vi "processamento_dos_dados_medios_de_caracterização.vi"() -> ()   [LabVIEW 2011]
uses:
  <vilib>/Analysis/NI_AALPro.lvlib
  <vilib>/Analysis/polynomials.llb/1D Polynomial Evaluation (DBL).vi
panel:
  out "Regressão Linear":string
  out "Coeficiente de Determinação":dbl
  out "Força aplicada (N)":dbl[](array[numeric])
  out "Força calculada \n(N)":dbl[](array[numeric])
  out "Coeficientes da Regressão":dbl[](array[numeric])
  out "Tensão e Força do Sinal":cluster{"Y":dbl[], "Y":dbl[]}[](graph)
  out "Tensão elétrica \nmedida (mV/V)":dbl[](array[numeric])
  # "PROGRAMA PARA O PROCESSAMENTO DOS DADOS \nDO PROCEDIMENTO DE CARACTERIZAÇÃO"
  # "CONVERSÃO DE TENSÃO ELÉTRICA (mV/V) PARA FORÇA (N)"
  # "Desenvolvido por Eloi Antonio Triaca"
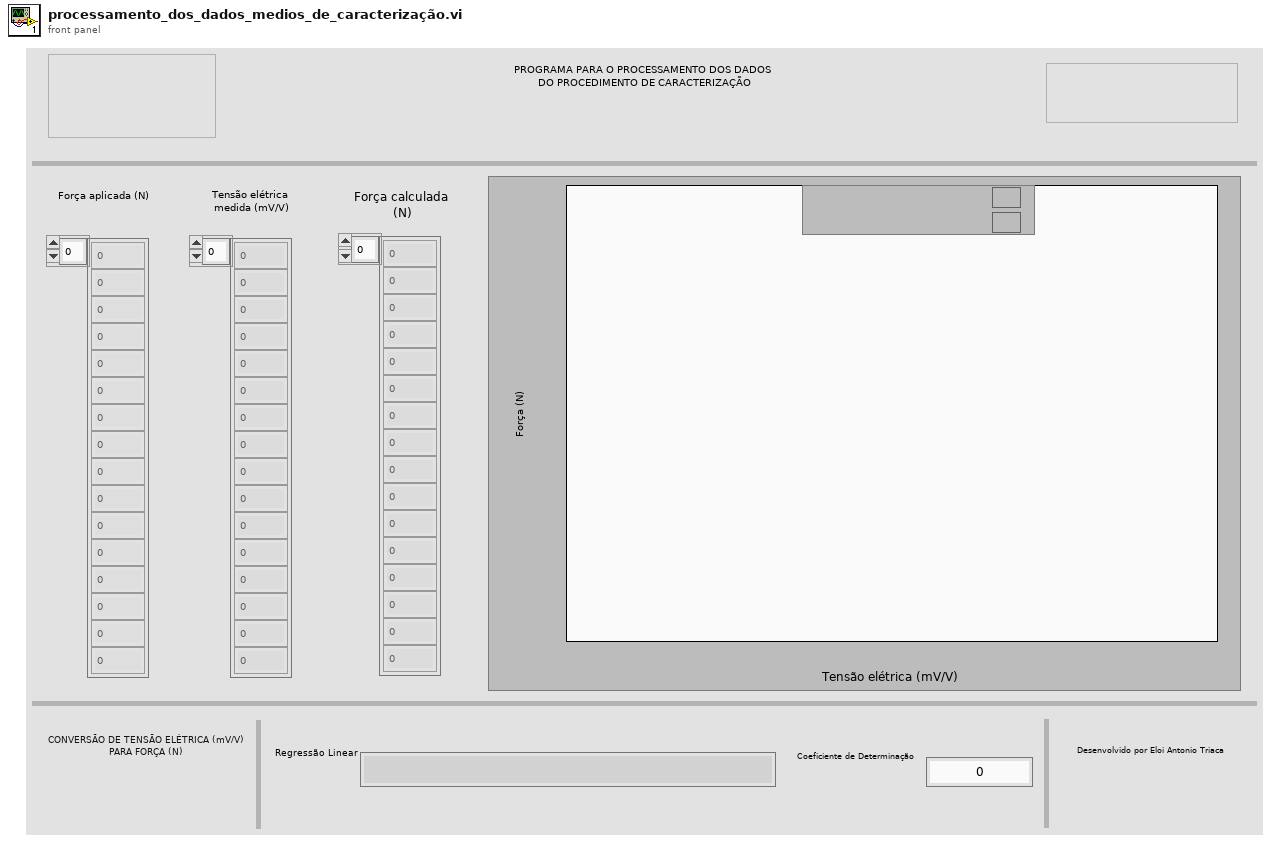
[diagram p1: front panel]
types:
  T1 = cluster{"Best Polynomial Fit":dbl[], "array":dbl[]}
  T2 = cluster{"Best Polynomial Fit":dbl[], "array":dbl[]}[]
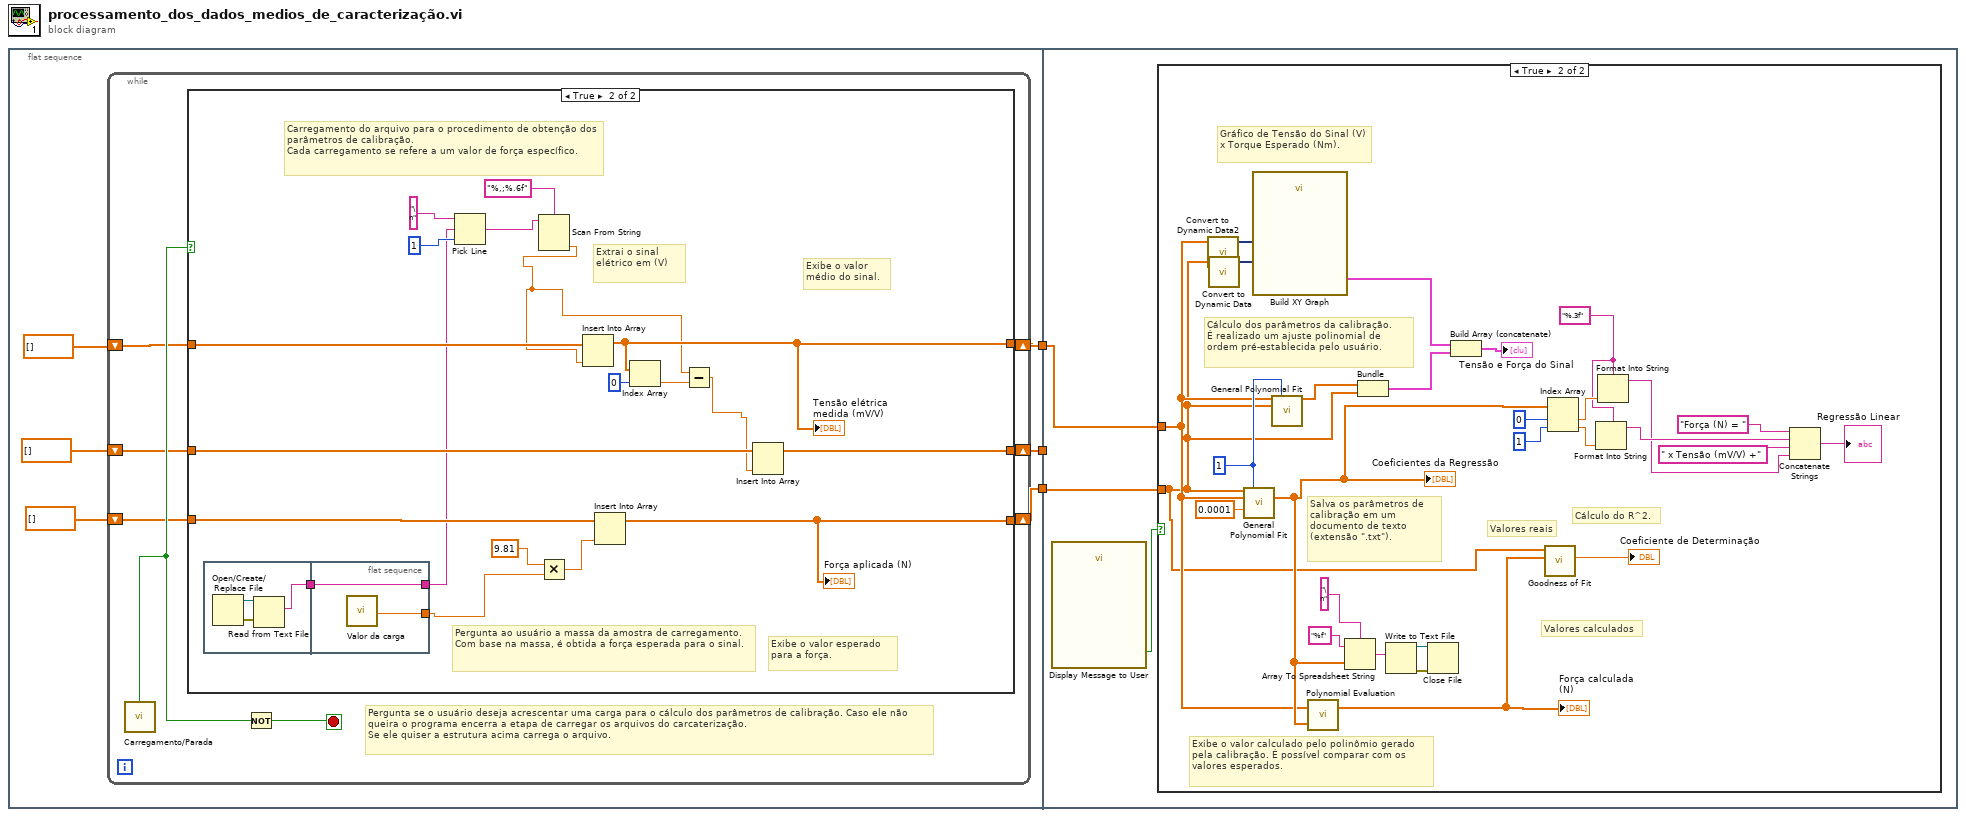
[diagram p0: block diagram]
diagram:
  n1 = flat-sequence {
    tunnel: [w8] -> w3
    tunnel: [w4] -> w2
    tunnel: [w6] -> w1
    tunnel: w3 -> [w45]
    tunnel: w2 -> [w47]
    tunnel: w1 -> [_]
    frame #0 {
      n2 = while {
        shift-right: [w14] -> w8
        shift-left: dbl[] [] ("array") -> [w15]
        shift-right: [w12] -> w6
        shift-left: dbl[] [] ("array") -> [w13]
        shift-right: [w10] -> w4
        shift-left: dbl[] [] ("array") -> [w11]
        stop <- w17 stop-if-true
        # "Pergunta se o usuário deseja acrescentar uma carga para o cálculo dos parâmetros de calibração. Caso ele não queira o programa encerra a etapa de carregar os arquivos do carcaterização.\nSe ele quiser a estrutura acima carrega o arquivo."
        n3 = call "Carregamento/Parada"() -> ("Carregar"=w16:bool)  [unwired: 18 in, 1 out]
        n4 = case shown="True" w16 {
          tunnel: w15 -> [w20 w35]
          tunnel: [w20 w22] -> w14
          tunnel: w13 -> [w19 w32]
          tunnel: [w19 w31] -> w12
          tunnel: w11 -> [w18 w28]
          tunnel: [w18 w26] -> w10
          frame False {
          }
          frame True {
            # "Exibe o valor esperado para a força."
            # "Exibe o valor médio do sinal."
            # "Carregamento do arquivo para o procedimento de obtenção dos parâmetros de calibração.\nCada carregamento se refere a um valor de força específico."
            # "Pergunta ao usuário a massa da amostra de carregamento. Com base na massa, é obtida a força esperada para o sinal."
            # "Extrai o sinal elétrico em (V)"
            n5 = flat-sequence {
              tunnel: [w40] -> w25
              tunnel: [w44] -> w23
              tunnel: w25 -> [w44]
              tunnel: [w43] -> w24
              frame #0 {
                n6 = Open/Create/Replace File() -> (refnum out=w41:refnum<file>, error out=w42:errorcluster)  [unwired: 6 in, 1 out]
                n7 = Read from Text File(file (use dialog)=w41, error in=w42) -> (text=w40:string)  [unwired: 2 in, 3 out]
              }
              frame #1 {
                n8 = call "Valor da carga"() -> ("Carga"=w43:dbl)  [unwired: 17 in, 2 out]
              }
            }
            n9 = Pick Line(string ("")="\n", multi-line string=w23, line index=1) -> (output string=w37:string)
            n10 = Scan From String(format string="%,;%.6f", input string=w37) -> (output 1=w21:dbl)  [unwired: 3 in, 3 out]
            n11 = Multiply(x=9.81, y=w24) -> (x*y=w27:dbl)
            n12 = Insert Into Array(array=w35, new element=w21) -> (w22:dbl[])  [unwired: 1 in]
            "Tensão elétrica \nmedida (mV/V)" <- w22
            n13 = Insert Into Array(array=w28, new element=w27) -> (w26:dbl[])  [unwired: 1 in]
            "Força aplicada (N)" <- w26
            n14 = Index Array(array=w22, index=0) -> (element=w33:dbl)
            n15 = Subtract(x=w21, y=w33) -> (x-y=w30:dbl)
            n16 = Insert Into Array(array=w32, new element=w30) -> (w31:dbl[])  [unwired: 1 in]
          }
        }
        n17 = Not(x=w16) -> (.not. x?=w17:bool)
      }
    }
    frame #1 {
      n18 = call "Display Message to User"() -> ("OK"=w46:bool)  [unwired: 10 in, 1 out]
      n19 = case shown="True" w46 {
        tunnel: w45 -> [_ w54]
        tunnel: w47 -> [_ w50]
        frame False {
        }
        frame True {
          w48 = "%.3f" ("format string")
          w69 = 1 ("Ordem da regressão")
          # "Valores calculados"
          # "Cálculo do R^2."
          # "Valores reais"
          # "Salva os parâmetros de calibração em um documento de texto (extensão \".txt\")."
          # "Exibe o valor calculado pelo polinômio gerado pela calibração. É possível comparar com os valores esperados."
          # "Cálculo dos parâmetros da calibração. \nÉ realizado um ajuste polinomial de ordem pré-establecida pelo usuário."
          # "Gráfico de Tensão do Sinal (V) x Torque Esperado (Nm)."
          n20 = call "Convert to Dynamic Data2"("Array"=w54) -> ("Dynamic Data Type"=w51:dynamicdata)  [unwired: 3 in]
          n21 = call "Convert to Dynamic Data"("Array"=w50) -> ("Dynamic Data Type"=w52:dynamicdata)  [unwired: 3 in]
          n22 = call <vilib>:"General Polynomial Fit.vi"("Y"=w50, "polynomial order"=w69, "X"=w54, "tolerance"=0.0001) -> ("Polynomial Coefficients"=w55:dbl[])  [unwired: 8 in, 3 out]
          "Coeficientes da Regressão" <- w55
          n23 = call "Build XY Graph"("Y Input"=w52, "X Input"=w51) -> ("XY Graph"=w68:cluster{"Y":dbl[], "Y":dbl[]}[])  [unwired: 3 in, 6 out]
          n24 = call <vilib>:"General Polynomial Fit.vi"("Y"=w54, "polynomial order"=w69, "X"=w50) -> ("Best Polynomial Fit"=w49:dbl[])  [unwired: 9 in, 3 out]
          n25 = call-poly <vilib>:"Polynomial Evaluation.vi"("P(x)"=w55, "A"=w54) -> ("P(A)"=w53:dbl[])  [unwired: 1 out]
          "Força calculada \n(N)" <- w53
          n26 = Array To Spreadsheet String(delimiter (Tab)="\n", array=w55, 3:"%f" ("format string")) -> (spreadsheet string=w70:string)
          n27 = Bundle("Best Polynomial Fit"=w49, "array"=w50) -> (w67:T1)  [unwired: 1 in]
          n28 = Write to Text File(text=w70) -> (refnum out=w72:refnum<file>, error out=w71:errorcluster)  [unwired: 3 in, 1 out]
          n29 = Close File(refnum=w72, error in=w71) -> ()  [unwired: 2 out]
          n30 = Build Array (concatenate)(w68, w67) -> (→"Tensão e Força do Sinal":T2)
          n31 = call <vilib>:"Goodness of Fit.vi"("Best Fit"=w53, "Y"=w50) -> ("R-square"=→"Coeficiente de Determinação":dbl)  [unwired: 6 in, 3 out]
          n32 = Index Array(array=w55, index #1=0 ("index"), index #2=1 ("index")) -> (element #1=w62:dbl, element #2=w61:dbl)
          n33 = Format Into String(format string=w48, w61) -> (resulting string=w58:string)  [unwired: 2 in, 1 out]
          n34 = Format Into String(format string=w48, w62) -> (resulting string=w57:string)  [unwired: 2 in, 1 out]
          n35 = Concatenate Strings("Força (N) = ", w58, " x Tensão (mV/V) +", w57) -> (→"Regressão Linear":string)
        }
      }
    }
  }
